vi "CommonVIs_TwoButtonDialog.vi"(1 "message":string, 3 "yesButtonName":string="OK", 4 "noButtonName":string="Cancel", 5 "error in (no error)":errorcluster, 6 "WindowTitle":string, 7 "timeout(-1 ms) -1=infinity":i32=-1) -> (13 "timeOut":bool=TRUE, 16 "yesButtonPressed":bool, 19 "error out":errorcluster)   [LabVIEW 2020]
doc: "Displays a dialog box that contains a message and two buttons. <B>yesButtonName</B> and <B>noButtonName</B> are the names displayed on the buttons of the dialog box."
panel:
  in  "noButton":bool
  in  "yesButton":bool
  out "showMessage":string
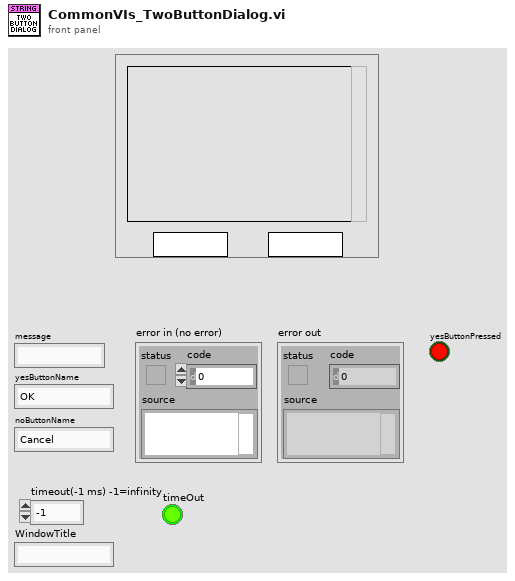
[diagram p1: front panel]
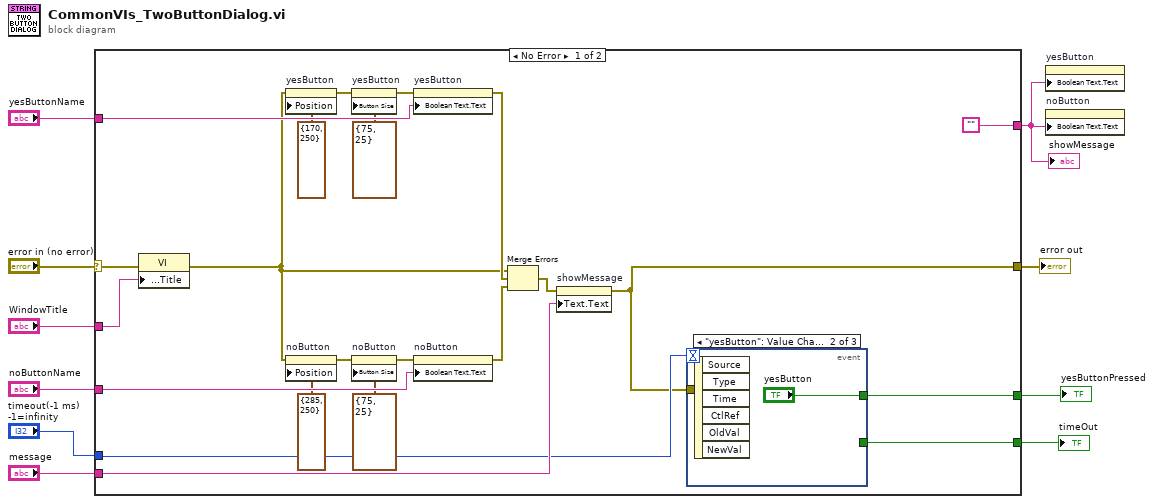
[diagram p0: block diagram]
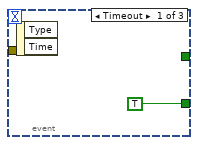
[diagram p2: hidden frame]
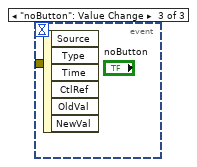
[diagram p3: hidden frame]
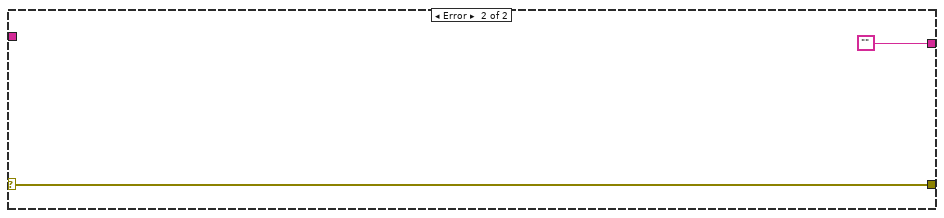
[diagram p4: hidden frame]
diagram:
  n1 = case shown="No Error" "error in (no error)" {
    selector: "error in (no error)" -> [w32 w36]
    tunnel: [w11 w36] -> w10
    tunnel: "noButtonName" -> [w31 _]
    tunnel: "yesButtonName" -> [w29 _]
    tunnel: ["" ""] -> w6
    tunnel: "message" -> [w28 _]
    tunnel: "timeout(-1 ms) -1=infinity" -> [w16 _]
    tunnel: [w15 _] -> w3
    tunnel: [w14 _] -> w2
    tunnel: "WindowTitle" -> [w13 _]
    frame No Error {
      n2 = property class="VI"(error in=w32, "Front Panel Window:Title"=w13) -> (error out=w12:errorcluster)  [unwired: 1 in, 1 out]
      n3 = property on="yesButton" class="Bool"(error in=w12, "Position"=cluster{"Left":i32, "Top":i32} {"Left"=170, "Top"=250}) -> (error out=w25:errorcluster)  [unwired: 1 in, 1 out]
      n4 = property on="noButton" class="Bool"(error in=w12, "Position"=cluster{"Left":i32, "Top":i32} {"Left"=285, "Top"=250}) -> (error out=w24:errorcluster)  [unwired: 1 in, 1 out]
      n5 = property on="yesButton" class="Bool"(error in=w25, "Button Size"=cluster{"Width":u32, "Height":u32} {"Width"=75, "Height"=25}) -> (error out=w26:errorcluster)  [unwired: 1 in, 1 out]
      n6 = property on="noButton" class="Bool"(error in=w24, "Button Size"=cluster{"Width":u32, "Height":u32} {"Width"=75, "Height"=25}) -> (error out=w23:errorcluster)  [unwired: 1 in, 1 out]
      n7 = property on="yesButton" class="Bool"(error in=w26, "Boolean Text.Text"=w29) -> (error out=w21:errorcluster)  [unwired: 1 in, 1 out]
      n8 = property on="noButton" class="Bool"(error in=w23, "Boolean Text.Text"=w31) -> (error out=w22:errorcluster)  [unwired: 1 in, 1 out]
      n9 = Merge Errors(w12, w21, w22) -> (w17:errorcluster)
      n10 = property on="showMessage" class="Str"(error in=w17, "Text.Text"=w28) -> (error out=w11:errorcluster)  [unwired: 1 in, 1 out]
      n11 = event shown="[1] \"yesButton\": Value Change" {
        selector: _ -> [_ _ _]
        dyn-events: _ -> [_ _ _]
        timeout: w16 -> [_ _ _]
        tunnel: [TRUE _ _] -> w15
        tunnel: [_ "yesButton" _] -> w14
        tunnel: w11 -> [_ _ _]
        event Timeout {
          n12 = event-data() -> ()  [unwired: 3 out]
        }
        event "yesButton": Value Change {
          n13 = event-data() -> ()  [unwired: 7 out]
        }
        event "noButton": Value Change {
          n14 = event-data() -> ()  [unwired: 7 out]
        }
      }
    }
    frame Error {
    }
  }
  "error out" <- w10
  "yesButtonPressed" <- w2
  "showMessage" <- w6
  "timeOut" <- w3
  n15 = property on="yesButton" class="Bool"("Boolean Text.Text"=w6) -> ()  [unwired: 2 in, 2 out]
  n16 = property on="noButton" class="Bool"("Boolean Text.Text"=w6) -> ()  [unwired: 2 in, 2 out]
